vi "Test Remove Test Class from Suite.vi"(8 "error in (no error)":errorcluster, 11 "LUnit Test Suite Tests in":refnum<class "LUnit Test Suite Tests.lvclass">) -> (0 "error out":errorcluster, 3 "LUnit Test Suite Tests out":refnum<class "LUnit Test Suite Tests.lvclass">)   [LabVIEW 2020, in "LUnit Test Suite Tests.lvclass"]
uses:
  LUnit Test Suite Tests.lvclass
  C:/Program Files (x86)/National Instruments/LabVIEW 2020/vi.lib/Astemes/LUnit/Core/LUnit Test Case/Test Case.lvclass
  Test Doubles/Test Case Test Double/Test Case Test Double.lvclass
  <vilib>/Astemes/LUnit/Core/LUnit Test Case/Test Case.lvclass/Test Case.ctl
  <vilib>/Astemes/LUnit/Core/LUnit Test Case/Private/Append Fail Result.vi
  <vilib>/Astemes/LUnit/Core/LUnit Test Case/Private/Append Pass Result.vi
  <vilib>/Astemes/LUnit/Core/LUnit Test Case/Private/Run In UI.vi
  <vilib>/Utility/error.llb/Clear Errors.vi
  source/LUnit Test Suite.lvclass
  C:/git/astemes-lunit/source/Core/Runnable/Runnable.lvclass
  <vilib>/Astemes/LUnit/Core/LUnit Test Case/Test Case.lvclass
panel:
  out "List of Runnables":string[](array[string])
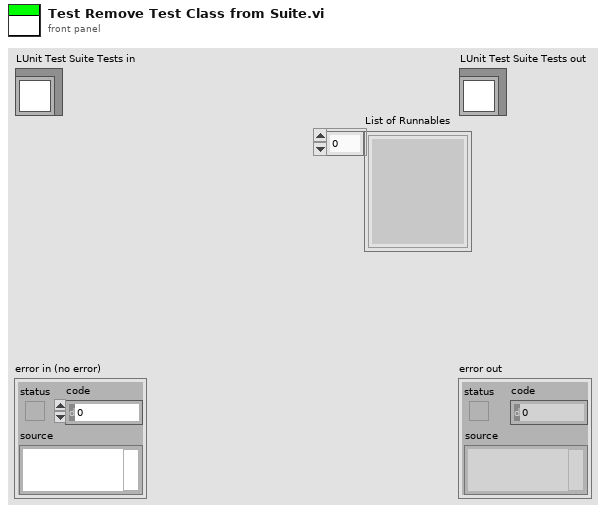
[diagram p1: front panel]
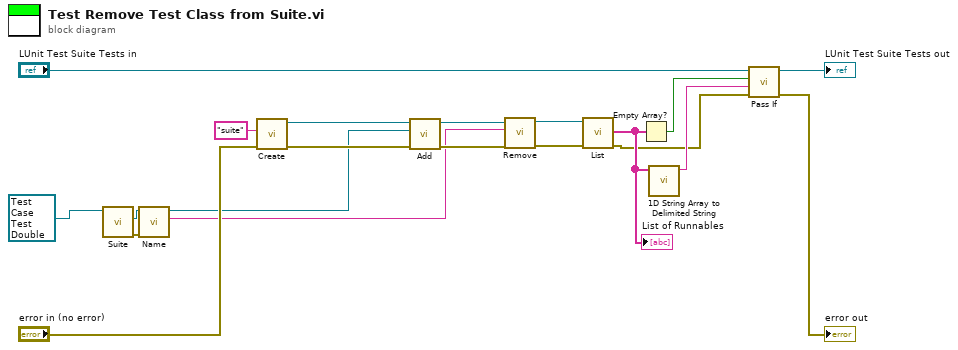
[diagram p0: block diagram]
diagram:
  n1 = call-dynamic "Suite.vi"("LUnit Test Case In"=refnum<class "Test Case Test Double.lvclass"> refnum ("Test Case Test Double.lvclass")) -> ("error out"=w4:errorcluster, "LUnit Test Suite Out"=w3:refnum<class "LUnit Test Suite.lvclass">)  [unwired: 8 in, 1 out]
  n2 = call-dynamic "Name.vi"("error in (no error)"=w4, "LUnit Test Suite in"=w3) -> ("Name"=w1:string, "LUnit Test Suite out"=w2:refnum<class "LUnit Test Suite.lvclass">)  [unwired: 7 in, 1 out]
  n3 = call "Create.vi"("error in (no error)"="error in (no error)", "Suite Name"="suite") -> ("error out"=w18:errorcluster, "LUnit Test Suite Out"=w19:refnum<class "LUnit Test Suite.lvclass">)  [unwired: 8 in]
  n4 = call "Add.vi"("error in (no error)"=w18, "Runnable"=w2, "LUnit Test Suite In"=w19) -> ("error out"=w16:errorcluster, "LUnit Test Suite Out"=w17:refnum<class "LUnit Test Suite.lvclass">)  [unwired: 7 in]
  n5 = call "Remove.vi"("error in (no error)"=w16, "Test to Remove"=w1, "LUnit Test Suite In"=w17) -> ("error out"=w14:errorcluster, "LUnit Test Suite Out"=w15:refnum<class "LUnit Test Suite.lvclass">)  [unwired: 7 in]
  n6 = call "List.vi"("error in (no error)"=w14, "LUnit Test Suite In"=w15) -> ("error out"=w7:errorcluster, "List of Runnables"=w9:string[])  [unwired: 8 in]
  "List of Runnables" <- w9
  n7 = Empty Array?(array=w9) -> (empty?=w10:bool)
  n8 = call <vilib>:"1D String Array to Delimited String.vi"("string array"=w9) -> ("delimited string"=w8:string)  [unwired: 10 in]
  n9 = call <vilib>:"Pass If.vi"("error in (no error)"=w7, "Message"=w8, "Pass?"=w10, "LUnit Test Case In"="LUnit Test Suite Tests in") -> ("error out"=→"error out":errorcluster, "LUnit Test Case Out"=→"LUnit Test Suite Tests out":refnum<class "LUnit Test Suite Tests.lvclass">)  [unwired: 6 in]
